vi "ActionVIOnLoad.vi"(8 "error in (no error)":errorcluster, 11 "Device Item Ref in":T1 format="%.0x") -> (0 "error out":errorcluster, 3 "Device Item Ref out":T1 format="%.0x")   [LabVIEW 2027, in "Embedded Data Logger System Explorer.lvlib"]
uses:
  Embedded Data Logger System Explorer.lvlib
  <vilib>/NI VeriStand/Custom Device API/Custom Device Item Ref.ctl
  <vilib>/NI VeriStand/Custom Device API/Custom Device API.lvlib
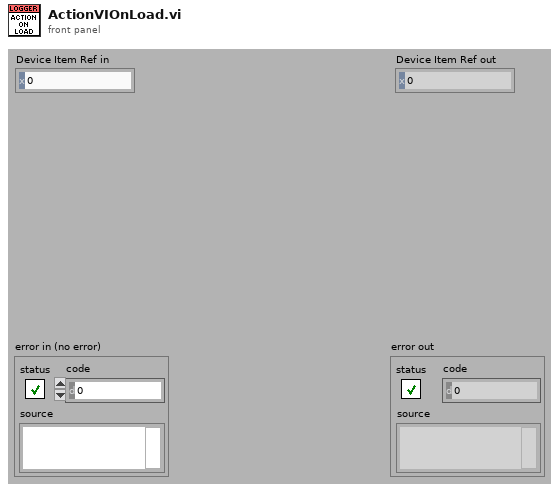
[diagram p1: front panel]
types:
  T1 = typedef "Custom Device API.lvlib/Custom Device Item Ref.ctl" = u64
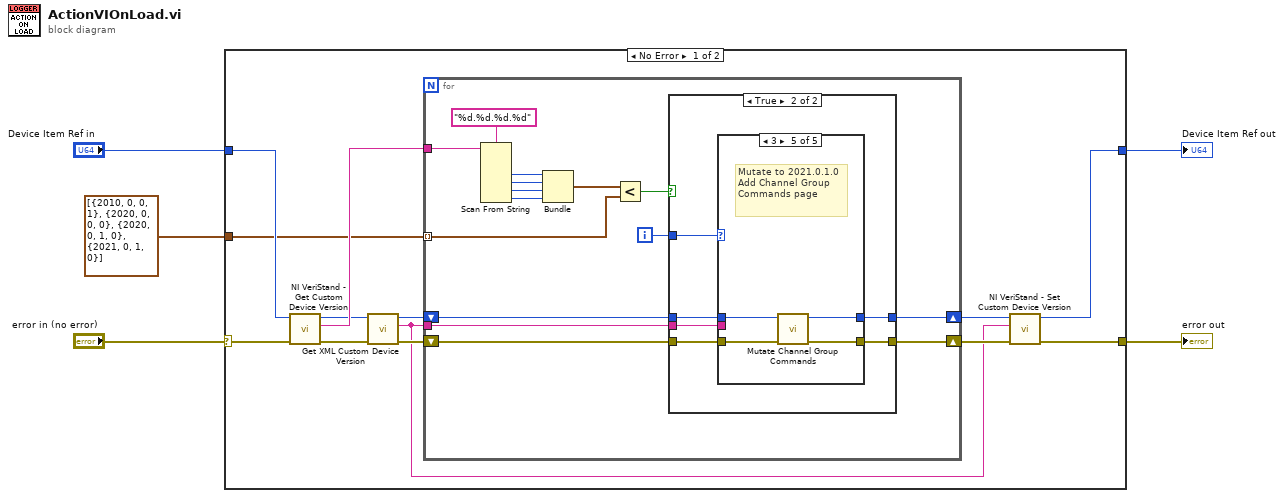
[diagram p0: block diagram]
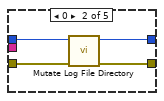
[diagram p4: hidden frame]
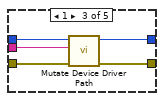
[diagram p5: hidden frame]
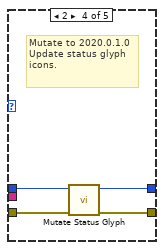
[diagram p6: hidden frame]
diagram:
  n1 = case shown="No Error" "error in (no error)" {
    selector: "error in (no error)" -> [w18 w62]
    tunnel: [w15 w62] -> w4
    tunnel: [w16 w61] -> w3
    tunnel: "Device Item Ref in" -> [w17 w61]
    tunnel: cluster{i32, i32, i32, i32}[] [{2010, 0, 0, 1}, {2020, 0, 0, 0}, {2020, 0, 1, 0}, {2021, 0, 1, 0}] -> [w13 _]
    frame No Error {
      n2 = call <vilib>:"NI VeriStand - Get Custom Device Version.vi"("error in (no error)"=w18, "Device Ref in"=w17) -> ("error out"=w8:errorcluster, "Value"=w14:string, "Device Ref out"=w10:T1)  [unwired: 7 in]
      n3 = call "Get XML Custom Device Version.vi"("error in (no error)"=w8, "Device Ref in"=w10) -> ("error out"=w7:errorcluster, "Version"=w6:string, "Device Ref out"=w9:T1)  [unwired: 7 in]
      n4 = for {
        tunnel: w14 -> [w31]
        tunnel: w13 -> [w30] mode=indexing
        shift-right: [w23] -> w12
        shift-left: w9 -> [w33]
        shift-right: [w22] -> w11
        shift-left: w7 -> [w32]
        tunnel: w6 -> [w19]
        i -> [w20]
        n5 = Scan From String(format string="%d.%d.%d.%d", input string=w31) -> (output 1=w28:i32, output 2=w27:i32, output 3=w26:i32, output 4=w25:i32)  [unwired: 6 in, 3 out]
        n6 = Bundle(w28, w27, w26, w25) -> (w24:cluster{i32, i32, i32, i32})  [unwired: 1 in]
        n7 = Less?(x=w24, y=w30) -> (x < y?=w21:bool)
        n8 = case shown="True" w21 {
          tunnel: w33 -> [w35 w41]
          tunnel: w32 -> [w34 w40]
          tunnel: [w35 w39] -> w23
          tunnel: [w34 w38] -> w22
          tunnel: w20 -> [_ w37]
          tunnel: w19 -> [_ w36]
          frame False {
          }
          frame True {
            n9 = case shown="3" w37 {
              tunnel: w41 -> [w43 w47 w52 w56 w58]
              tunnel: w40 -> [w42 w46 w50 w55 w60]
              tunnel: [w43 w45 w51 w53 w57] -> w39
              tunnel: [w42 w44 w49 w54 w59] -> w38
              tunnel: w36 -> [_ _ w48 _ _]
              frame Default {
              }
              frame 0 {
                n10 = call "Mutate Log File Directory.vi"("error in (no error)"=w46, "Device Ref in"=w47) -> ("error out"=w44:errorcluster, "Device Ref out"=w45:T1)  [unwired: 8 in]
              }
              frame 1 {
                n11 = call "Mutate Device Driver Path.vi"("error in (no error)"=w50, "Version"=w48, "Device Ref in"=w52) -> ("error out"=w49:errorcluster, "Device Ref out"=w51:T1)  [unwired: 7 in]
              }
              frame 2 {
                # "Mutate to 2020.0.1.0\nUpdate status glyph  icons."
                n12 = call "Mutate Status Glyph.vi"("error in"=w55, "device in"=w56) -> ("error out"=w54:errorcluster, "device out"=w53:T1)  [unwired: 8 in]
              }
              frame 3 {
                # "Mutate to 2021.0.1.0\nAdd Channel Group Commands page"
                n13 = call "Mutate Channel Group Commands.vi"("error in"=w60, "device in"=w58) -> ("error out"=w59:errorcluster, "device out"=w57:T1)  [unwired: 8 in]
              }
            }
          }
        }
      }
      n14 = call <vilib>:"NI VeriStand - Set Custom Device Version.vi"("error in (no error)"=w11, "Value"=w6, "Device Ref in"=w12) -> ("error out"=w15:errorcluster, "Device Ref out"=w16:T1)  [unwired: 7 in]
    }
    frame Error {
    }
  }
  "error out" <- w4
  "Device Item Ref out" <- w3
